vi "Get ClassName.vi"(8 "error in (no error)":errorcluster, 11 "Message in":refnum<class "Message.lvclass">) -> (0 "error out":errorcluster, 2 "Class Name":string, 3 "Message out":refnum<class "Message.lvclass">)   [LabVIEW 2013, in "LapDog.Messaging.v3.lvlib" / "Message.lvclass"]
doc: "Returns the <b>class name</b> (not message name) of the object on the wire at runtime. Class Name does not return the fully qualified name of the object nor the .lvclass extension.\n\nThis method executes regardless of the error in state."
uses:
  Message.lvclass
  <vilib>/regexp/Match Regular Expression.xnode
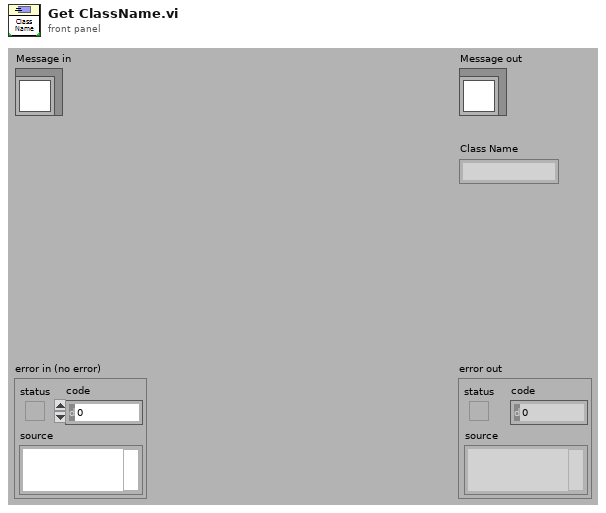
[diagram p1: front panel]
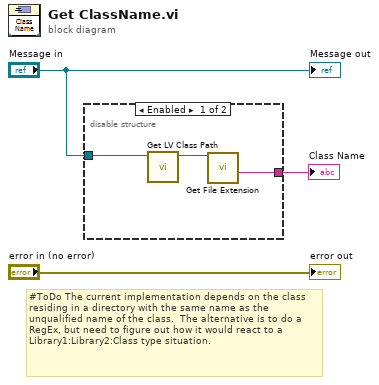
[diagram p0: block diagram]
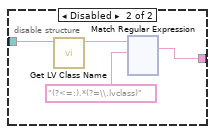
[diagram p2: hidden frame]
diagram:
  # "#ToDo The current implementation depends on the class residing in a directory with the same name as the unqualified name of the class.  The alternative is to do a RegEx, but need to figure out how it would react to a Library1:Library2:Class type situation."
  n1 = disable-structure shown="Enabled" {
    disable-tunnel: [w6 w7] -> w3
    disable-tunnel: "Message in" -> [w5 w10]
    frame Enabled {
      n2 = call <vilib>:"Get LV Class Path.vi"("object"=w5) -> ("class path"=w4:path)  [unwired: 1 in, 9 out]
      n3 = call <vilib>:"Get File Extension.vi"("file"=w4) -> ("filename without extension"=w6:string)  [unwired: 1 in, 9 out]
    }
    frame Disabled {
      n4 = call <vilib>:"Get LV Class Name.vi"("object"=w10) -> ("class name"=w8:string)  [unwired: 9 in, 1 out]
      n5 = xnode "Match Regular Expression"("input string"=w8, "regular expression"="(?<=:).*(?=\\.lvclass)") -> ("whole match"=w7:string)  [unwired: 4 in, 4 out]
    }
  }
  "Class Name" <- w3
  "error out" <- "error in (no error)"
  "Message out" <- "Message in"
